vi "Main.vi"(8 "error in":errorcluster, 11 "Table in":refnum<class "Table.lvclass">) -> (0 "error out":errorcluster, 3 "Table out":refnum<class "Table.lvclass">)   [LabVIEW 2021, in "Table.lvclass"]
doc: "The <b>Queued Message Handler</b> of the Worker that owns this VI."
uses:
  Table.lvclass
  Table.lvclass/Table.ctl
  Initialization Data.ctl
  Philosopher/Philosopher.lvclass
  Hungry.ctl
  Fork.ctl
  <vilib>/addons/_Workers/Library/Case Label.ctl
  <vilib>/addons/_Workers/Library/Workers.lvlib
  Philosopher/Response Cases.ctl
  <vilib>/Utility/miscctls.llb/LVRectTypeDef.ctl
  Philosopher/Initialization Data.ctl
  6539f85e-2771-4448-8291-956c93914d8b.vi
panel:
  in  "The End":bool
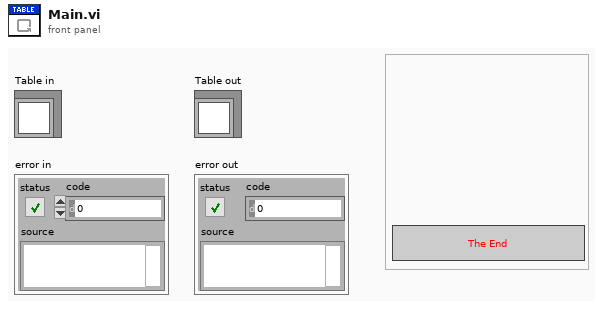
[diagram p1: front panel]
types:
  T1 = typedef "Table.lvclass/Initialization Data.ctl" = cluster{"# Philosophers":i32}
  T2 = typedef "Philosopher.lvclass/Initialization Data.ctl" = cluster{"Response Cases":T3, "ID":i32, "FP.PanelBounds":T5}
  T3 = typedef "Philosopher.lvclass/Response Cases.ctl" = cluster{"Hungry":T4, "Done":T4}
  T4 = typedef "Workers.lvlib/Case Label.ctl" = string
  T5 = typedef "LVRectTypeDef.ctl" = cluster{"Left":i16, "Top":i16, "Right":i16, "Bottom":i16}
  T6 = typedef "Table.lvclass/Fork.ctl" = enum16{"FREE", "IN USE"}
  T7 = typedef "Table.lvclass/Hungry.ctl" = enum16{"NO", "YES"}
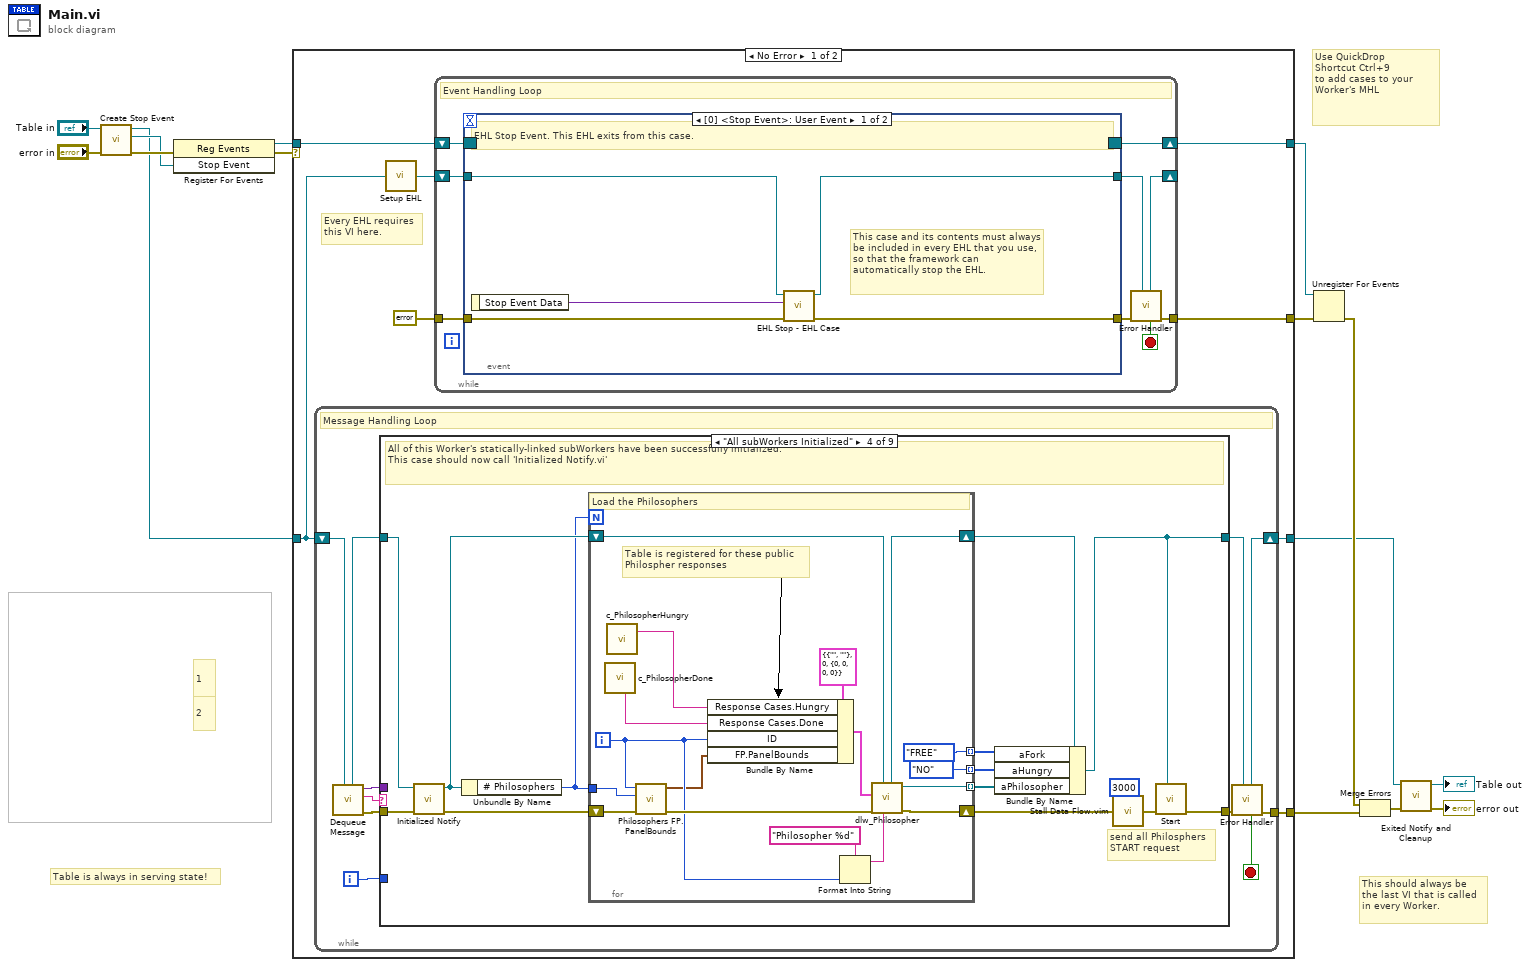
[diagram p0: block diagram]
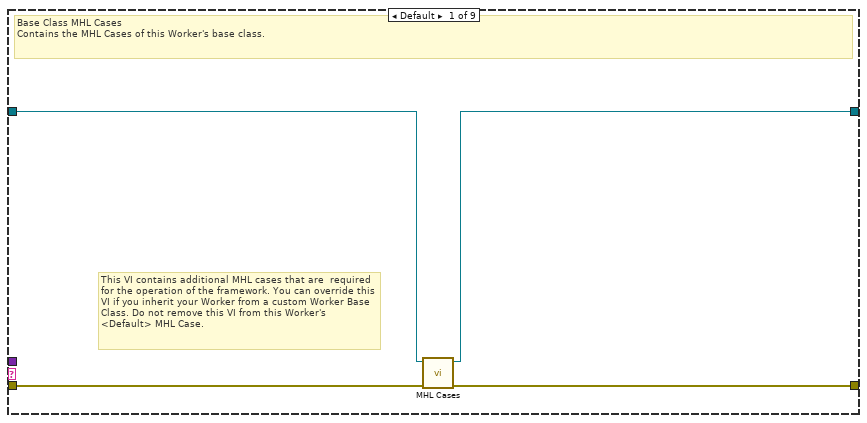
[diagram p2: hidden frame]
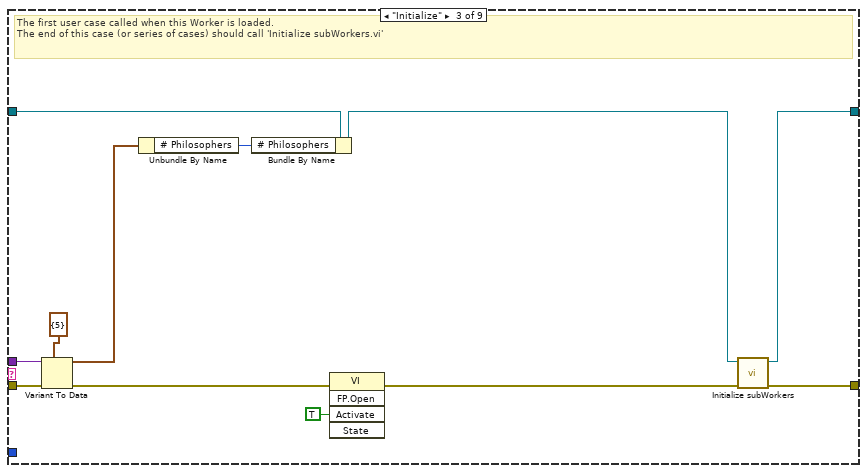
[diagram p4: hidden frame]
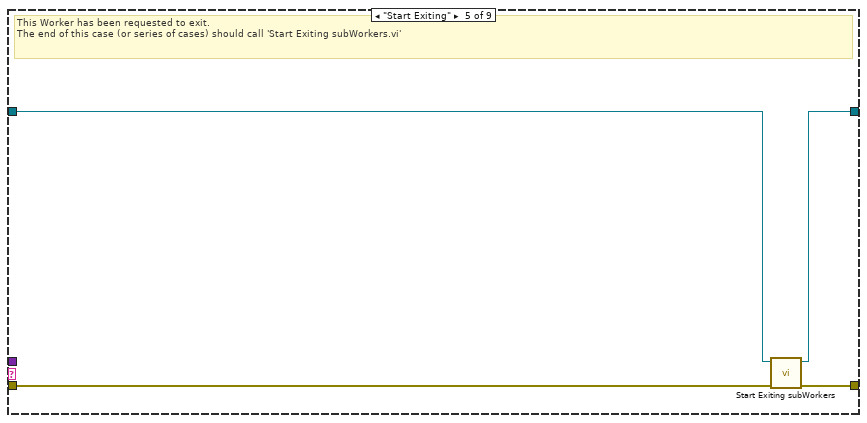
[diagram p5: hidden frame]
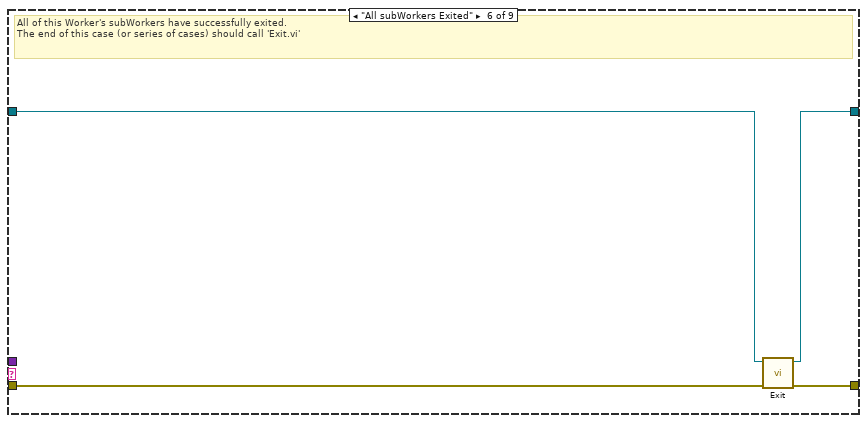
[diagram p6: hidden frame]
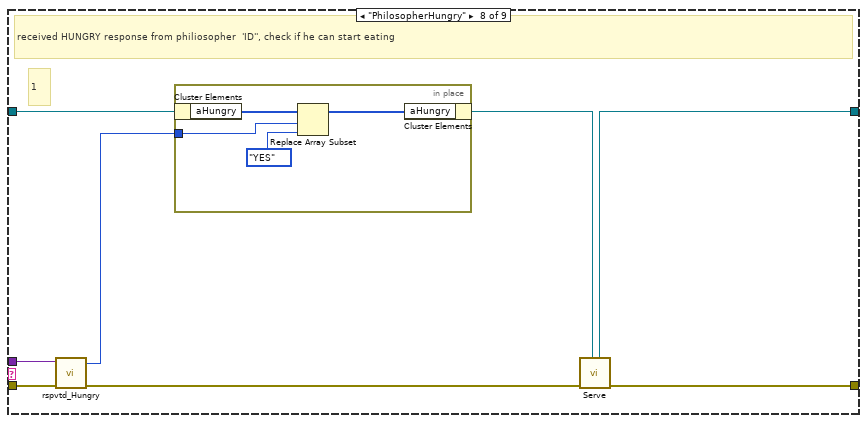
[diagram p8: hidden frame]
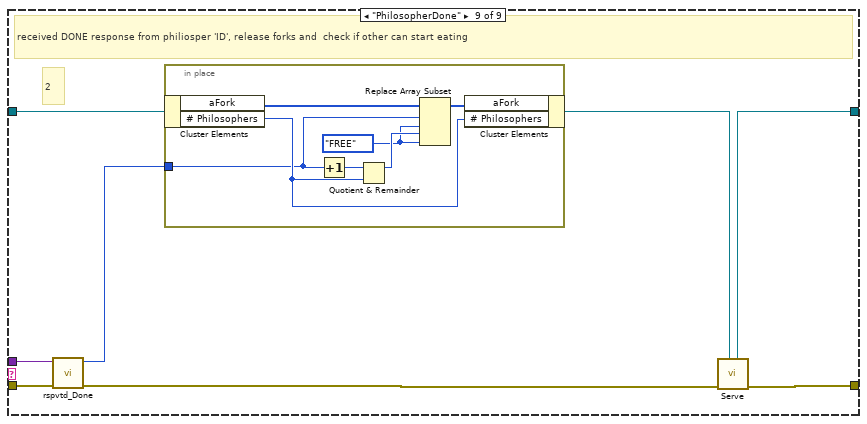
[diagram p9: hidden frame]
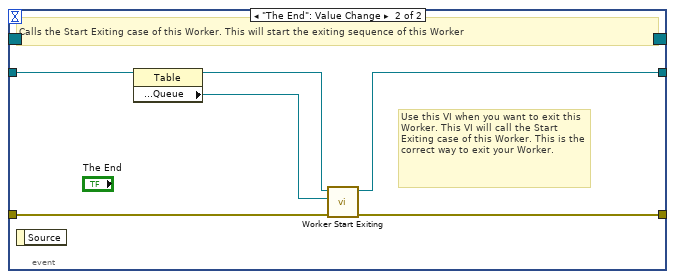
[diagram p10: hidden frame]
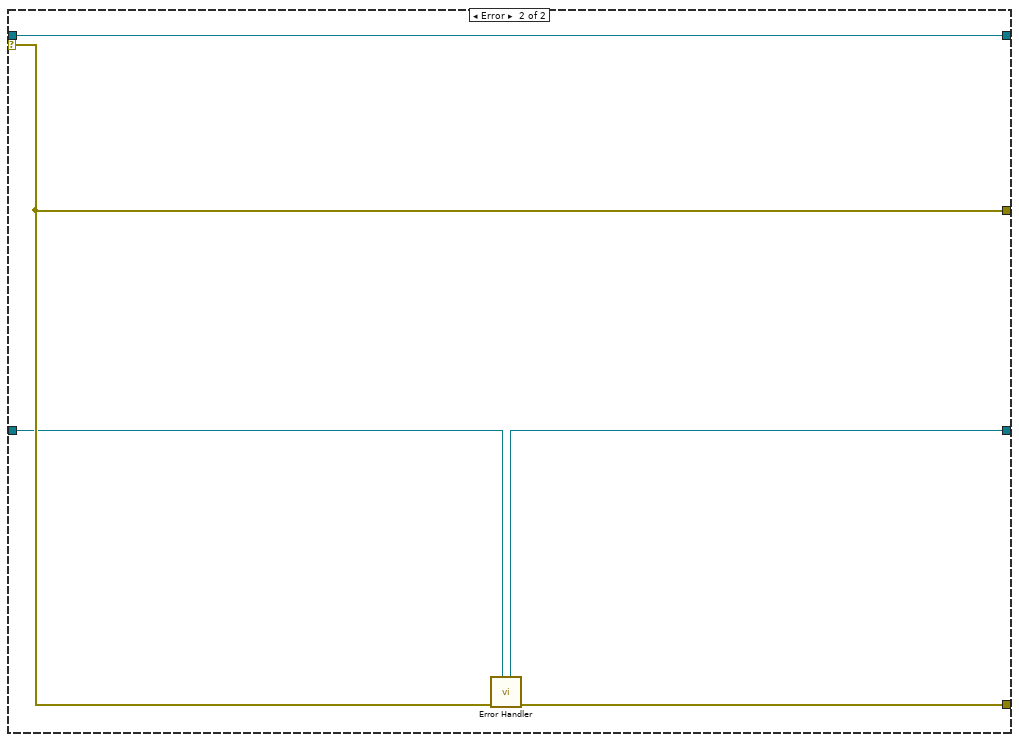
[diagram p11: hidden frame]
diagram:
  # "2"
  # "1"
  # "Table is always in serving state!"
  # "Use QuickDrop\nShortcut Ctrl+9\nto add cases to your\nWorker's MHL"
  # "This should always be the last VI that is called in every Worker."
  n1 = call-dynamic "Create Stop Event.vi"("error in"="error in", "Worker"="Table in") -> ("error out"=w10:errorcluster, "Stop Event"=w7:refnum<user-event>, "Worker out"=w4:refnum<class "Table.lvclass">)  [unwired: 7 in]
  n2 = register-events(error in=w10, w7) -> (reference out=w9:refnum<event-registration>, error out=w1:errorcluster)  [unwired: 1 in]
  n3 = case shown="No Error" w1 {
    tunnel: w4 -> [w18 w142]
    tunnel: [w16 w143] -> w8
    tunnel: w9 -> [w23 w144]
    tunnel: [w20 w145] -> w14
    tunnel: [w22 w144] -> w13
    tunnel: [w17 w141] -> w11
    selector: w1 -> [_ w145]
    frame No Error {
      # "Every EHL requires\nthis VI here."
      n4 = while {
        shift-right: [w32] -> w17
        shift-left: w18 -> [w34]
        tunnel: [w33] -> w16
        i -> [w25]
        stop <- w26 stop-if-true
        # "Message Handling Loop"
        n5 = call-dynamic "Dequeue Message.vi"("Worker"=w34) -> ("error out"=w31:errorcluster, "Case out"=w27:string, "Data out"=w24:variant, "Worker out"=w29:refnum<class "Table.lvclass">)  [unwired: 6 in, 1 out]
        n6 = case "Worker MHL Case Structure (DO NOT CHANGE LABEL NAME)" shown="\"All subWorkers Initialized\"" w27 {
          tunnel: w31 -> [w38 w39 w50 w65 w84 w91 w93 w100 w113]
          tunnel: [w37 w39 w52 w57 w87 w90 w93 w97 w110] -> w30
          tunnel: w29 -> [w36 w40 w49 w66 w85 w89 w92 w99 w109]
          tunnel: [w35 w40 w51 w56 w86 w88 w92 w95 w107] -> w28
          tunnel: w25 -> [_ _ _ _ _ _ _ _ _]
          tunnel: w24 -> [_ _ w48 _ _ _ _ w101 w112]
          frame Default {
            # "This VI contains additional MHL cases that are  required for the operation of the framework. You can override this VI if you inherit your Worker from a custom Worker Base Class. Do not remove this VI from this Worker's <Default> MHL Case."
            # "Base Class MHL Cases\nContains the MHL Cases of this Worker's base class."
            n7 = call-dynamic "MHL Cases.vi"("error in"=w38, "Worker in"=w36) -> ("error out"=w37:errorcluster, "Worker out"=w35:refnum<class "Table.lvclass">)  [unwired: 8 in]
          }
          frame "------------ FRAMEWORK CASES -----------" {
            # "Start of Workers Framework Cases"
          }
          frame "Initialize" {
            # "The first user case called when this Worker is loaded.\nThe end of this case (or series of cases) should call 'Initialize subWorkers.vi'"
            n8 = Variant To Data(error in=w50, type=T1 {"# Philosophers"=5} ("Initialization Data"), Variant=w48) -> (data=w47:T1, error out=w43:errorcluster)
            n9 = Unbundle By Name(w47) -> ("# Philosophers"=w45:i32)
            n10 = Bundle By Name(cluster=w49, "# Philosophers"=w45) -> (w44:refnum<class "Table.lvclass">)
            n11 = invoke on="Invoke Node" class="VI" method="FP.Open"(error in=w43, "Activate"=TRUE ("Activate?")) -> (error out=w42:errorcluster)  [unwired: 3 in, 4 out]
            n12 = call-dynamic "Initialize subWorkers.vi"("error in"=w42, "Worker"=w44) -> ("error out"=w52:errorcluster, "dup Worker out"=w51:refnum<class "Table.lvclass">)  [unwired: 8 in]
          }
          frame "All subWorkers Initialized" {
            # "send all Philosphers\nSTART request"
            # "All of this Worker's statically-linked subWorkers have been successfully initialized.\nThis case should now call 'Initialized Notify.vi'"
            n13 = call-dynamic "Initialized Notify.vi"("error in"=w65, "Worker"=w66) -> ("error out"=w64:errorcluster, "dup Worker out"=w63:refnum<class "Table.lvclass">)  [unwired: 8 in]
            n14 = Unbundle By Name(w63) -> ("# Philosophers"=w55:i32)
            n15 = for {
              N: w55 -> [_]
              shift-right: [w83] -> w58
              shift-left: w64 -> [w74]
              tunnel: [w79] -> w61 mode=indexing
              tunnel: [Fork."FREE" ("Fork")] -> w60 mode=indexing
              tunnel: [Hungry."NO" ("Hungry")] -> w62 mode=indexing
              shift-right: [w80] -> w59
              shift-left: w63 -> [w77]
              tunnel: w55 -> [w71]
              i -> [w72]
              # "Table is registered for these public \nPhilospher responses"
              # "Load the Philosophers"
              n16 = call "c_PhilosopherDone.vi"() -> ("Case Label"=w75:T4)  [unwired: 1 in]
              n17 = call "c_PhilosopherHungry.vi"() -> ("Case Label"=w67:T4)  [unwired: 1 in]
              n18 = call "Philosophers FP.PanelBounds.vi"("error in"=w74, "# Philosophers"=w71, "Philospoher"=w72) -> ("error out"=w73:errorcluster, "Location chair"=w68:T5)  [unwired: 7 in]
              n19 = Bundle By Name(cluster=T2 {"Response Cases"={"Hungry"="", "Done"=""}, "ID"=0, "FP.PanelBounds"={"Left"=0, "Top"=0, "Right"=0, "Bottom"=0}} ("Initialization Data"), "Response Cases.Hungry"=w67, "Response Cases.Done"=w75, "ID"=w72, "FP.PanelBounds"=w68) -> (w70:T2)
              n20 = Format Into String(format string="Philosopher %d", w72) -> (resulting string=w81:string)  [unwired: 2 in, 1 out]
              n21 = call "dlw_Philosopher.vi"("Worker Alias"=w81, "Caller in"=w77, "error in"=w73, "Initialization Data"=w70) -> ("error out"=w83:errorcluster, "Philosopher out"=w79:refnum<class "Philosopher.lvclass">, "dup Caller out"=w80:refnum<class "Table.lvclass">)  [unwired: 5 in]
            }
            n22 = Bundle By Name(cluster=w59, "aFork"=w60, "aHungry"=w62, "aPhilosopher"=w61) -> (w56:refnum<class "Table.lvclass">)
            n23 = call "Stall Data Flow.vim"("value in"=w58, "milliseconds to wait"=u32 3000) -> ("value out"=w54:errorcluster)  [unwired: 1 out]
            n24 = call "Start.vi"("Table in"=w56, "error in"=w54) -> ("error out"=w57:errorcluster)  [unwired: 8 in, 1 out]
          }
          frame "Start Exiting" {
            # "This Worker has been requested to exit. \nThe end of this case (or series of cases) should call 'Start Exiting subWorkers.vi'"
            n25 = call-dynamic "Start Exiting subWorkers.vi"("error_in"=w84, "Worker"=w85) -> ("error out"=w87:errorcluster, "dup Worker out"=w86:refnum<class "Table.lvclass">)  [unwired: 8 in]
          }
          frame "All subWorkers Exited" {
            # "All of this Worker's subWorkers have successfully exited. \nThe end of this case (or series of cases) should call 'Exit.vi'"
            n26 = call-dynamic "Exit.vi"("error_in"=w91, "Worker"=w89) -> ("error out"=w90:errorcluster, "dup Worker out"=w88:refnum<class "Table.lvclass">)  [unwired: 8 in]
          }
          frame "------------- RESPONSE CASES --------------" {
            # "Start of Workers Response Cases"
          }
          frame "PhilosopherHungry" {
            # "1"
            # "received HUNGRY response from philiosopher  'ID'', check if he can start eating"
            n27 = call "rspvtd_Hungry.vi"("error in"=w100, "Data in"=w101) -> ("error out"=w98:errorcluster, "ID"=w94:i32)  [unwired: 8 in]
            n28 = in-place {
              in-place-border: w94 -> [w103]
              n29 = in-place-cluster #1(w99) -> ("aHungry"=w105:T7[])
              n30 = Replace Array Subset(array=w105, new element=Hungry."YES" ("new element/subarray"), index=w103) -> (w104:T7[])
              n31 = in-place-cluster #1("aHungry"=w104) -> (w96:refnum<class "Table.lvclass">)
            }
            n32 = call "Serve.vi"("Table in"=w96, "error in"=w98) -> ("error out"=w97:errorcluster, "Table out"=w95:refnum<class "Table.lvclass">)  [unwired: 8 in]
          }
          frame "PhilosopherDone" {
            # "2"
            # "received DONE response from philiosper 'ID', release forks and  check if other can start eating"
            n33 = call "rspvtd_Done.vi"("error in"=w113, "Data in"=w112) -> ("error out"=w111:errorcluster, "ID"=w106:i32)  [unwired: 8 in]
            n34 = in-place {
              in-place-border: w106 -> [w114]
              w115 = Fork."FREE" ("Fork")
              n35 = in-place-cluster #2(w109) -> ("aFork"=w118:T6[], "# Philosophers"=w116:i32)
              n36 = Increment(x=w114) -> (x+1=w120:i32)
              n37 = Quotient & Remainder(x=w120, y=w116) -> (x-y*floor(x/y)=w119:i32)  [unwired: 1 out]
              n38 = Replace Array Subset(array=w118, new element #1=w115, index #1=w114, new element #2=w115, index #2=w119) -> (w117:T6[])
              n39 = in-place-cluster #2("aFork"=w117, "# Philosophers"=w116) -> (w108:refnum<class "Table.lvclass">)
            }
            n40 = call "Serve.vi"("Table in"=w108, "error in"=w111) -> ("error out"=w110:errorcluster, "Table out"=w107:refnum<class "Table.lvclass">)  [unwired: 8 in]
          }
        }
        n41 = call-dynamic "Error Handler.vi"("Worker"=w28, "error_in"=w30) -> ("error out"=w33:errorcluster, "Stop Loop"=w26:bool, "Worker out"=w32:refnum<class "Table.lvclass">)  [unwired: 7 in]
      }
      n42 = call-dynamic "Setup EHL.vi"("Worker"=w18) -> ("Worker out"=w19:refnum<class "Table.lvclass">)  [unwired: 14 in]
      n43 = while "Event Handling Loop" {
        shift-right: [w129] -> w22
        shift-left: w23 -> [w128]
        tunnel: [w124] -> w20
        tunnel: errorcluster {"status"=FALSE, "code"=0, "source"=""} ("error constant") -> [w126]
        shift-right: [w122] -> _
        shift-left: w19 -> [w127]
        stop <- w121 stop-if-true
        # "Event Handling Loop"
        n44 = event shown="[0] <Stop Event>: User Event" {
          selector: w128 -> [_ _]
          dyn-events: [_ _] -> w129
          timeout: _ -> [_ _]
          tunnel: [w133 w139] -> w125
          tunnel: w126 -> [w134 w138]
          tunnel: w127 -> [w132 w140]
          tunnel: [w131 w136] -> w123
          event User Event {
            # "This case and its contents must always be included in every EHL that you use, so that the framework can automatically stop the EHL."
            # "EHL Stop Event. This EHL exits from this case."
            n45 = event-data() -> ("Stop Event Data"=w130:variant)  [unwired: 1 in]
            n46 = call-dynamic "EHL Stop - EHL Case.vi"("error in"=w134, "Stop Event Data"=w130, "Worker"=w132) -> ("error out"=w133:errorcluster, "Worker out"=w131:refnum<class "Table.lvclass">)  [unwired: 7 in]
          }
          event "The End": Value Change {
            # "Use this VI when you want to exit this Worker. This VI will call the Start Exiting case of this Worker. This is the correct way to exit your Worker."
            # "Calls the Start Exiting case of this Worker. This will start the exiting sequence of this Worker"
            n47 = event-data() -> ()  [unwired: 1 in, 1 out]
            n48 = property class="Table"(reference=w140) -> (reference out=w137:refnum<class "Table.lvclass">, "Accessors:Read:Public API:Queue"=w135:refnum<class "Message Queue.lvclass">)  [unwired: 1 in, 1 out]
            n49 = call-dynamic "Worker Start Exiting.vi"("error_in"=w138, "Message Queue"=w135, "Worker"=w137) -> ("error out"=w139:errorcluster, "dup Worker out"=w136:refnum<class "Table.lvclass">)  [unwired: 7 in]
          }
        }
        n50 = call-dynamic "Error Handler.vi"("Worker"=w123, "error_in"=w125) -> ("error out"=w124:errorcluster, "Stop Loop"=w121:bool, "Worker out"=w122:refnum<class "Table.lvclass">)  [unwired: 7 in]
      }
    }
    frame Error {
      n51 = call-dynamic "Error Handler.vi"("Worker"=w142, "error_in"=w145) -> ("error out"=w143:errorcluster, "Worker out"=w141:refnum<class "Table.lvclass">)  [unwired: 7 in, 1 out]
    }
  }
  n52 = Unregister For Events(event registration refnum=w13, error in=w14) -> (error out=w15:errorcluster)
  n53 = Merge Errors(w15, w8) -> (w12:errorcluster)
  n54 = call-dynamic "Exited Notify and Cleanup.vi"("error_in"=w12, "Worker"=w11) -> ("error out"=→"error out":errorcluster, "dup Worker out"=→"Table out":refnum<class "Table.lvclass">)  [unwired: 8 in]
